vi "labview project.vi"() -> ()   [LabVIEW 2020]
uses:
  <vilib>/MakerHub/LINX/Public/Sensors/Accelerometer/MPU60X0/DeviceAddresses.ctl
  <vilib>/MakerHub/LINX/Public/Sensors/Accelerometer/MPU60X0/Clock Source.ctl
  <vilib>/MakerHub/LINX/Public/Sensors/Accelerometer/MPU60X0/GyroFullScaleRanges.ctl
  <vilib>/MakerHub/LINX/Public/Utilities/Open Serial.vi
  <vilib>/Analysis/Matrix/Numeric/Conversions/Matrix To Array - RM.vi
  <vilib>/MakerHub/LINX/Public/Peripherals/PWM/PWM Set Duty Cycle N Chans.vi
  <vilib>/MakerHub/LINX/LMH-LINX.lvlib
  <vilib>/MakerHub/LINX/Public/Sensors/Accelerometer/MPU60X0/MPU60X0.lvlib
  <vilib>/Analysis/Matrix/NI_Matrix.lvlib
panel:
  out "Vitesse":i16(graph)
  out "Angle":dbl(graph)
  out "pitch angle":dbl
  out "roll angle":dbl
  in  "stop":bool
  out "Gyroscope Temperature":dbl
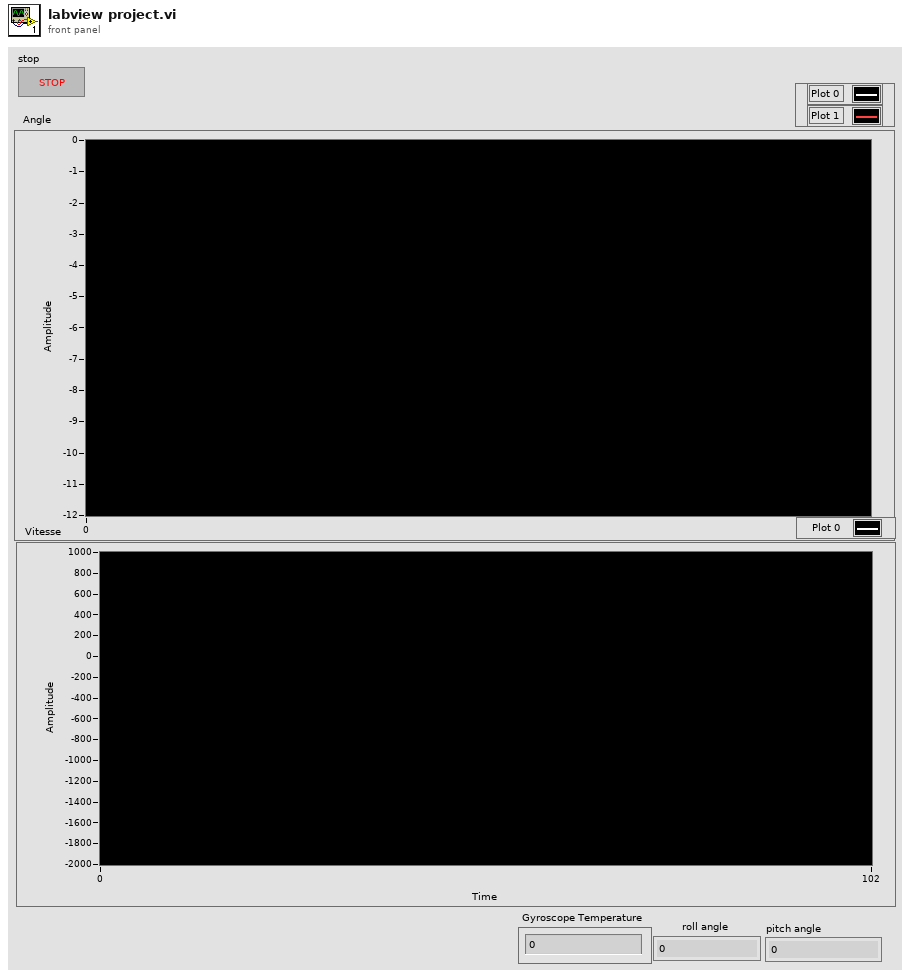
[diagram p1: front panel]
types:
  T1 = typedef "LMH-LINX.lvlib/MPU60X0.lvlib/GyroFullScaleRanges.ctl" = enum8{"±250 °/s", "±500 °/s", "±1000 °/s", "±2000 °/s"}
  T2 = typedef "LMH-LINX.lvlib/MPU60X0.lvlib/Clock Source.ctl" = enum8{"Internal 8MHz Osc", "PLL with X Gyro Ref", "PLL with Y Gyro Ref", "PLL with Z Gyro Ref", "PLL with ext 32.768 KHz Ref", "PLL with ext 19.2 MHz Ref", "Reserved", "Hold in reset"}
  T3 = typedef "LMH-LINX.lvlib/MPU60X0.lvlib/DeviceAddresses.ctl" = enum16{"0x68", "0x69"}
  T4 = typedef "LMH-LINX.lvlib/LINX Ref.ctl" = cluster{"IO":T5, "Interface":T6, "LINX Device Config":T7}
  T5 = typedef "LMH-LINX.lvlib/Platform.ctl" = enum16{"Remote", "Local"}
  T6 = typedef "LMH-LINX.lvlib/Interface.ctl" = enum16{"Serial", "TCP"}
  T7 = typedef "LMH-LINX.lvlib/Device.lvlib/LINX Device Config.ctl" = cluster{"Interface":T6, "COM Port":refnum<visa-resource-name>, "TCP Configuration":T8, "Device Family":u8, "Device ID":u8, "Device Name":string, "TCP Ref":refnum<k5>, "Channels":T9}
  T8 = typedef "LMH-LINX.lvlib/Device.lvlib/TCP Config.ctl" = cluster{"IP Address":string, "Port":u16}
  T9 = typedef "LMH-LINX.lvlib/Channels.ctl" = cluster{"DI":u8[], "DO":u8[], "AI":u8[], "AO":u8[], "PWM":u8[], "QE":u8[], "UART":u8[], "I2C 2":u8[], "SPI":u8[], "CAN":u8[], "Servo":u8[], "AI Ref (V)":dbl, "AI Resolution (Bits)":u8, "AO Ref (V)":dbl, "AO Resolution (Bits)":u8}
  T10 = cluster{"X Axis":i16, "Y Axis":i16, "Z Axis":i16}
  T11 = typedef "NI_Matrix.lvlib/RealMatrix.ctl" = dbl[][]
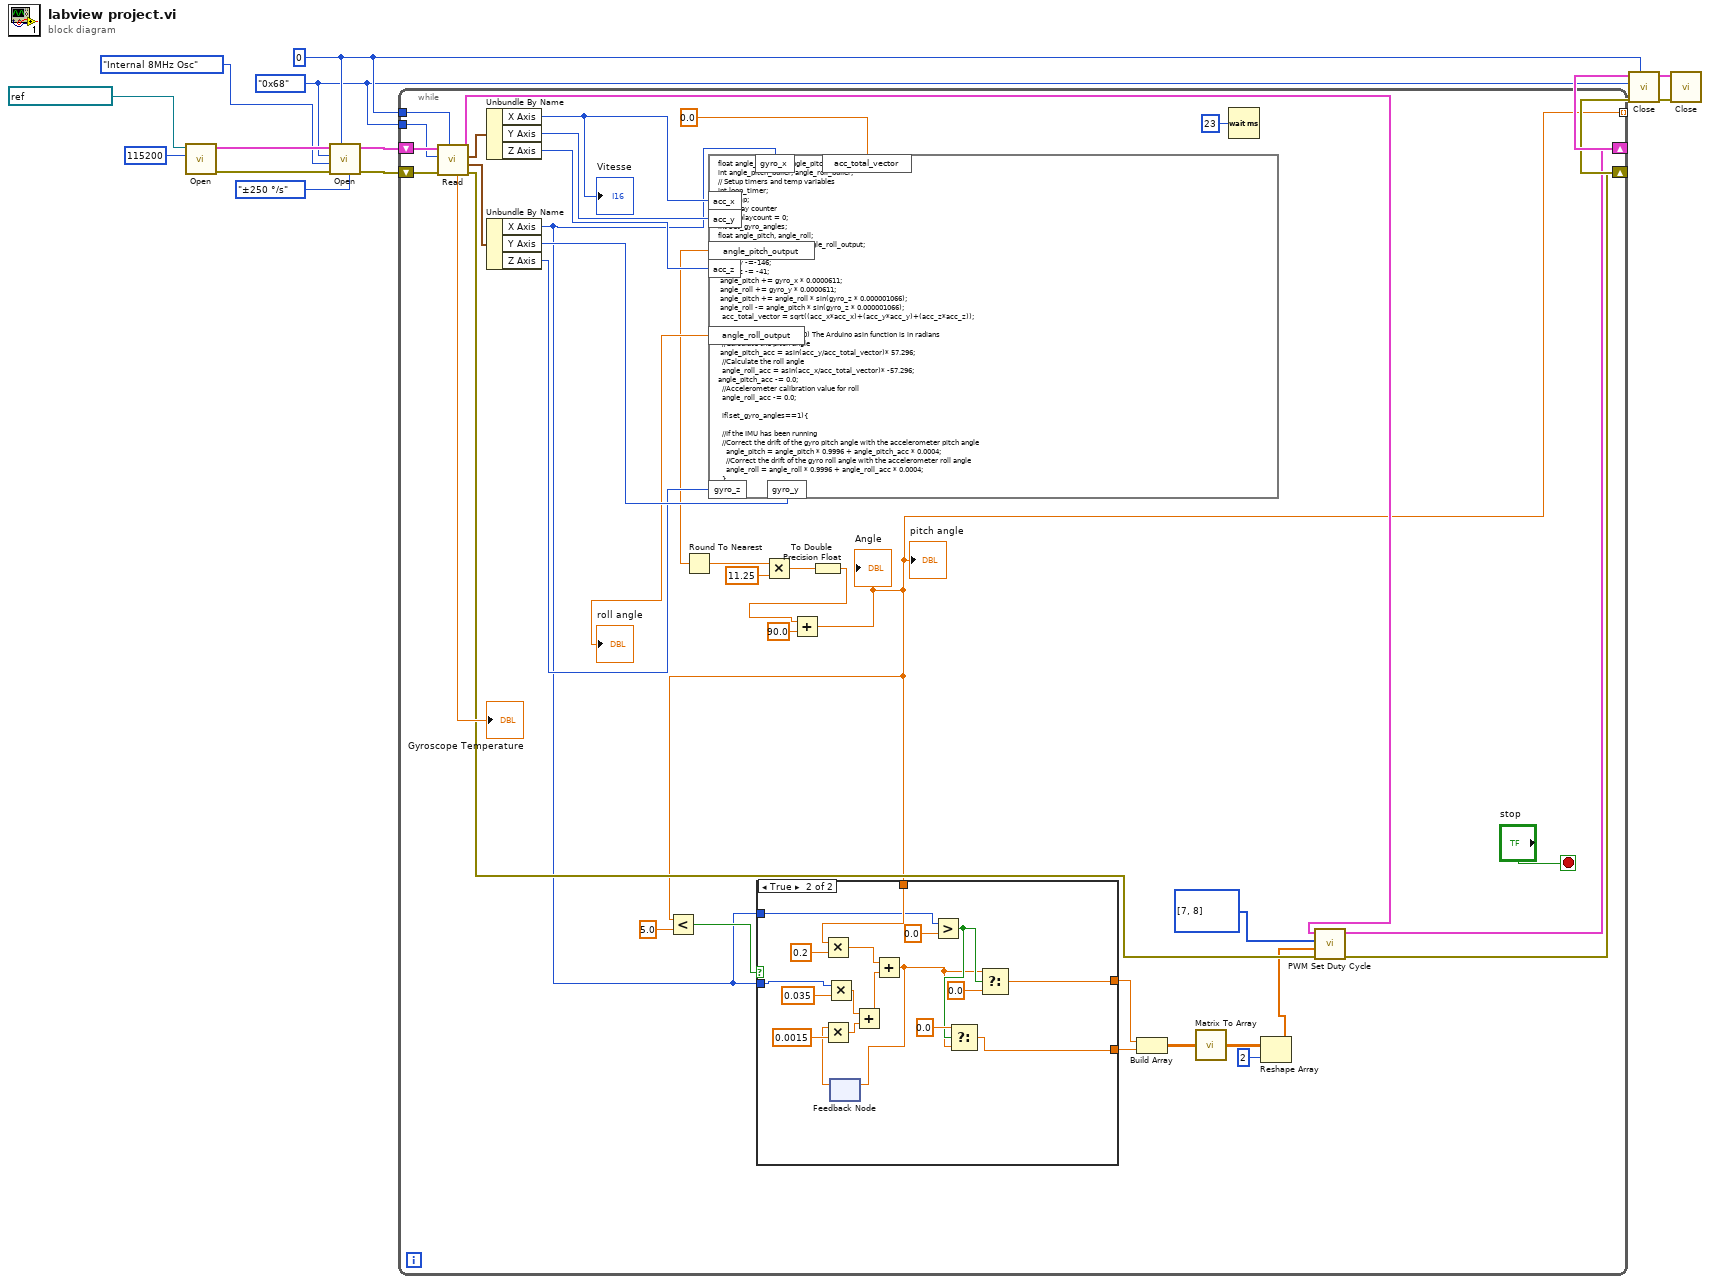
[diagram p0: block diagram]
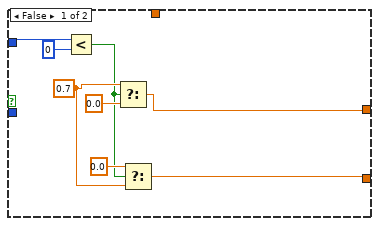
[diagram p2: hidden frame]
diagram:
  w6 = u8 0 ("I2C Channel")
  w2 = DeviceAddresses."0x68" ("I2C Slave Address")
  n1 = call-poly <vilib>:"Open.vi"("Baud Rate Override"=u32 115200, "Serial Port"=refnum<visa-resource-name> "ASRL53::INSTR") -> ("Error Out"=w10:errorcluster, "LINX Resource"=w14:T4)  [unwired: 7 in, 1 out]
  n2 = call <vilib>:"Open.vi"("Gyro Full Scale Range"=GyroFullScaleRanges."±250 °/s", "I2C Channel"=w6, "Error In"=w10, "Clock Source"=Clock_Source."Internal 8MHz Osc", "I2C Slave Address"=w2, "LINX Resource"=w14) -> ("Error Out"=w9:errorcluster, "LINX Resource"=w13:T4)  [unwired: 4 in]
  n3 = while {
    tunnel: w6 -> [w49]
    tunnel: w2 -> [w48]
    shift-right: [w29] -> w12
    shift-left: w13 -> [w51]
    shift-right: [w30] -> w8
    shift-left: w9 -> [w50]
    tunnel: [w20] -> _ mode=indexing
    stop <- "stop" stop-if-true
    n4 = call <vilib>:"Read.vi"("I2C Channel"=w49, "Error In"=w50, "I2C Slave Address"=w48, "LINX Resource"=w51) -> ("Error Out"=w32:errorcluster, "Gyro  Data (dps)"=w44:T10, "Acceleration Data (g)"=w45:T10, "LINX Resource"=w31:T4, "Temperature (°C)"=→"Gyroscope Temperature":dbl)  [unwired: 3 in]
    n5 = Unbundle By Name(w45) -> ("X Axis"=w37:i16, "Y Axis"=w40:i16, "Z Axis"=w39:i16)
    "Vitesse" <- w37
    n6 = Unbundle By Name(w44) -> ("X Axis"=w16:i16, "Y Axis"=w43:i16, "Z Axis"=w42:i16)
    n7 = formula code="float angle_roll_acc, angle_pitch_acc; \nint angle_pitch_buffer, angle_roll_buffer;\n// Setup timers and temp variables\nint loop_timer;\nint temp;\n// Display counter\nint displaycount = 0;\nint set_gyro_angles;\nfloat angle_pitch, angle_roll;\nfloat angle_pitch_output, angle_roll_output;\ngyro_x -= -121;                                                \n gyro_y -=-146;                                                \n gyro_z -= -41;                                                \n angle_pitch += gyro_x * 0.0000611;  \n angle_roll += gyro_y * 0.0000611; \n angle_pitch += angle_roll * sin(gyro_z * 0.000001066);             \n angle_roll -= angle_pitch * sin(gyro_z * 0.000001066);        \n  acc_total_vector = sqrt((acc_x*acc_x)+(acc_y*acc_y)+(acc_z*acc_z)); \n   \n  //57.296 = 1 / (3.142 / 180) The Arduino asin function is in radians\n  //Calculate the pitch angle\n angle_pitch_acc = asin(acc_y/acc_total_vector)* 57.296; \n  //Calculate the roll angle      \n  angle_roll_acc = asin(acc_x/acc_total_vector)* -57.296;                 \nangle_pitch_acc -= 0.0;\n  //Accelerometer calibration value for roll                                              \n  angle_roll_acc -= 0.0;                                               \n \n  if(set_gyro_angles==1){ \n  \n  //If the IMU has been running \n  //Correct the drift of the gyro pitch angle with the accelerometer pitch angle                      \n    angle_pitch = angle_pitch * 0.9996 + angle_pitch_acc * 0.0004; \n    //Correct the drift of the gyro roll angle with the accelerometer roll angle    \n    angle_roll = angle_roll * 0.9996 + angle_roll_acc * 0.0004;        \n  }\n  else{ \n    //IMU has just started  \n    //Set the gyro pitch angle equal to the accelerometer pitch angle                                                           \n    angle_pitch = angle_pitch_acc;\n    //Set the gyro roll angle equal to the accelerometer roll angle                                       \n    angle_roll = angle_roll_acc;\n    //Set the IMU started flag                                       \n    set_gyro_angles = 1;                                            \n  }\n  \n //To dampen the pitch and roll angles a complementary filter is used\n //Take 90% of the output pitch value and add 10% of the raw pitch value\nangle_pitch_output =angle_pitch_output * 0.9 + angle_pitch * 0.1; \n//Take 90% of the output roll value and add 10% of the raw roll value \nangle_roll_output = angle_roll_output * 0.9 + angle_roll * 0.1;\n//angle_pitch_output=11,25*angle_pitch_output; \n//angle_roll_output=11,25*angle_roll_output; \n\n//Wait until the loop_timer reaches 4000us (250Hz) before starting the next loop  \n   \n// Increment the display counter\ndisplaycount = displaycount +1;"("gyro_x"=w16, "gyro_y"=w43, "gyro_z"=w42, "acc_x"=w37, "acc_y"=w40, "acc_z"=w39, "acc_total_vector"=0.0) -> ("angle_pitch_output"=w35:dbl, "angle_roll_output"=→"roll angle":dbl)
    n8 = Round To Nearest(number=w35) -> (nearest integer value=w36:dbl)
    n9 = Multiply(x=w36, y=11.25) -> (x*y=w22:dbl)
    n10 = To Double Precision Float(number=w22) -> (double precision float=w19:dbl)
    n11 = Add(x=w19, y=90.0) -> (x+y=w20:dbl)
    "pitch angle" <- w20
    "Angle" <- w20
    n12 = Less?(x=w20, y=5.0) -> (x < y?=w33:bool)
    n13 = case shown="True" w33 {
      tunnel: w20 -> [_ w77]
      tunnel: w16 -> [_ w74]
      tunnel: [w55 w70] -> w18
      tunnel: [w56 w69] -> w17
      tunnel: w16 -> [w54 w66]
      frame False {
        w59 = 0.7
        n14 = Less?(x=w54, y=i16 0) -> (x < y?=w52:bool)
        n15 = Select(t=w59, s=w52, f=0.0) -> (s? t:f=w56:dbl)
        n16 = Select(t=0.0, s=w52, f=w59) -> (s? t:f=w55:dbl)
      }
      frame True {
        n17 = Multiply(x=w77, y=0.2) -> (x*y=w73:dbl)
        n18 = Multiply(x=w74, y=0.035) -> (x*y=w61:dbl)
        n19 = feedback #1() -> (w63:dbl)  [unwired: 1 in]
        n20 = Multiply(x=w63, y=0.0015) -> (x*y=w62:dbl)
        n21 = Add(x=w61, y=w62) -> (x+y=w60:dbl)
        n22 = Add(x=w73, y=w60) -> (x+y=w65:dbl)
        n23 = feedback-in #1(w65) -> ()
        n24 = Greater?(x=w66, y=0.0) -> (0:w67:bool)
        n25 = Select(t=0.0, s=w67, f=w65) -> (s? t:f=w70:dbl)
        n26 = Select(t=w65, s=w67, f=0.0) -> (s? t:f=w69:dbl)
      }
    }
    n27 = Build Array(w17, w18) -> (w26:T11)
    n28 = call-poly <vilib>:"Matrix To Array.vi"("Real Matrix"=w26) -> ("Real 2D Array"=w27:dbl[][])
    n29 = Wait (ms)(milliseconds to wait=u32 23) -> ()  [unwired: 1 out]
    n30 = Reshape Array(w27, 2 ("dimension size")) -> (w24:dbl[])
    n31 = call-poly <vilib>:"PWM Set Duty Cycle.vi"("Error In"=w32, "Duty Cycles"=w24, "PWM Channels"=u8[] [7, 8], "LINX Resource"=w31) -> ("Error Out"=w30:errorcluster, "LINX Resource"=w29:T4)  [unwired: 6 in]
  }
  n32 = call <vilib>:"Close.vi"("I2C Channel (0)"=w6, "Error In"=w8, "I2C Slave Address (0)"=w2, "LINX Resource"=w12) -> ("Error Out"=w7:errorcluster, "LINX Resource"=w11:T4)  [unwired: 6 in]
  n33 = call <vilib>:"Close.vi"("Error In"=w7, "LINX Resource"=w11) -> ()  [unwired: 9 in, 1 out]
